vi "DRAFT3.vi"() -> ()   [LabVIEW 2021]
uses:
  <vilib>/Analysis/3filter.llb/Butterworth Filter (DBL).vi
  <vilib>/Analysis/NI_AALBase.lvlib
  <vilib>/ptbypt/NI_PtbyPt.lvlib
panel:
  out "Array Size":u32
  out "Elapsed time in ms":u32
  in  "stop":bool
  in  "error in (no error)":errorcluster
  out "error out":errorcluster
  in  "loop 1":i32
  out "Waveform Graph 6":dynamicdata(graph)
  out "Waveform Graph 5":dynamicdata(graph)
  out "Waveform Graph 4":dynamicdata(graph)
  out "Waveform Graph 3":dbl[](graph)
  out "Waveform Graph 2":dynamicdata(graph)
  in  "Boolean":bool
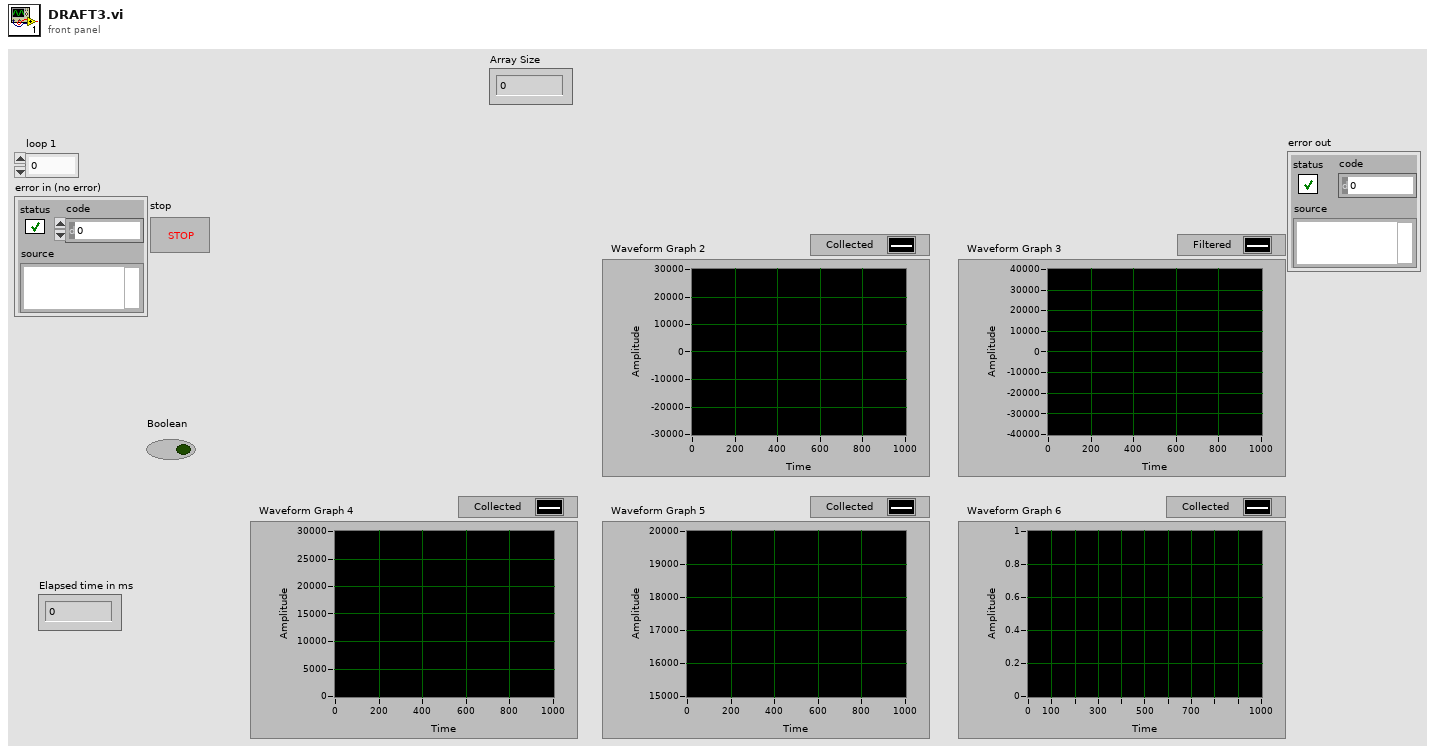
[diagram p1: front panel]
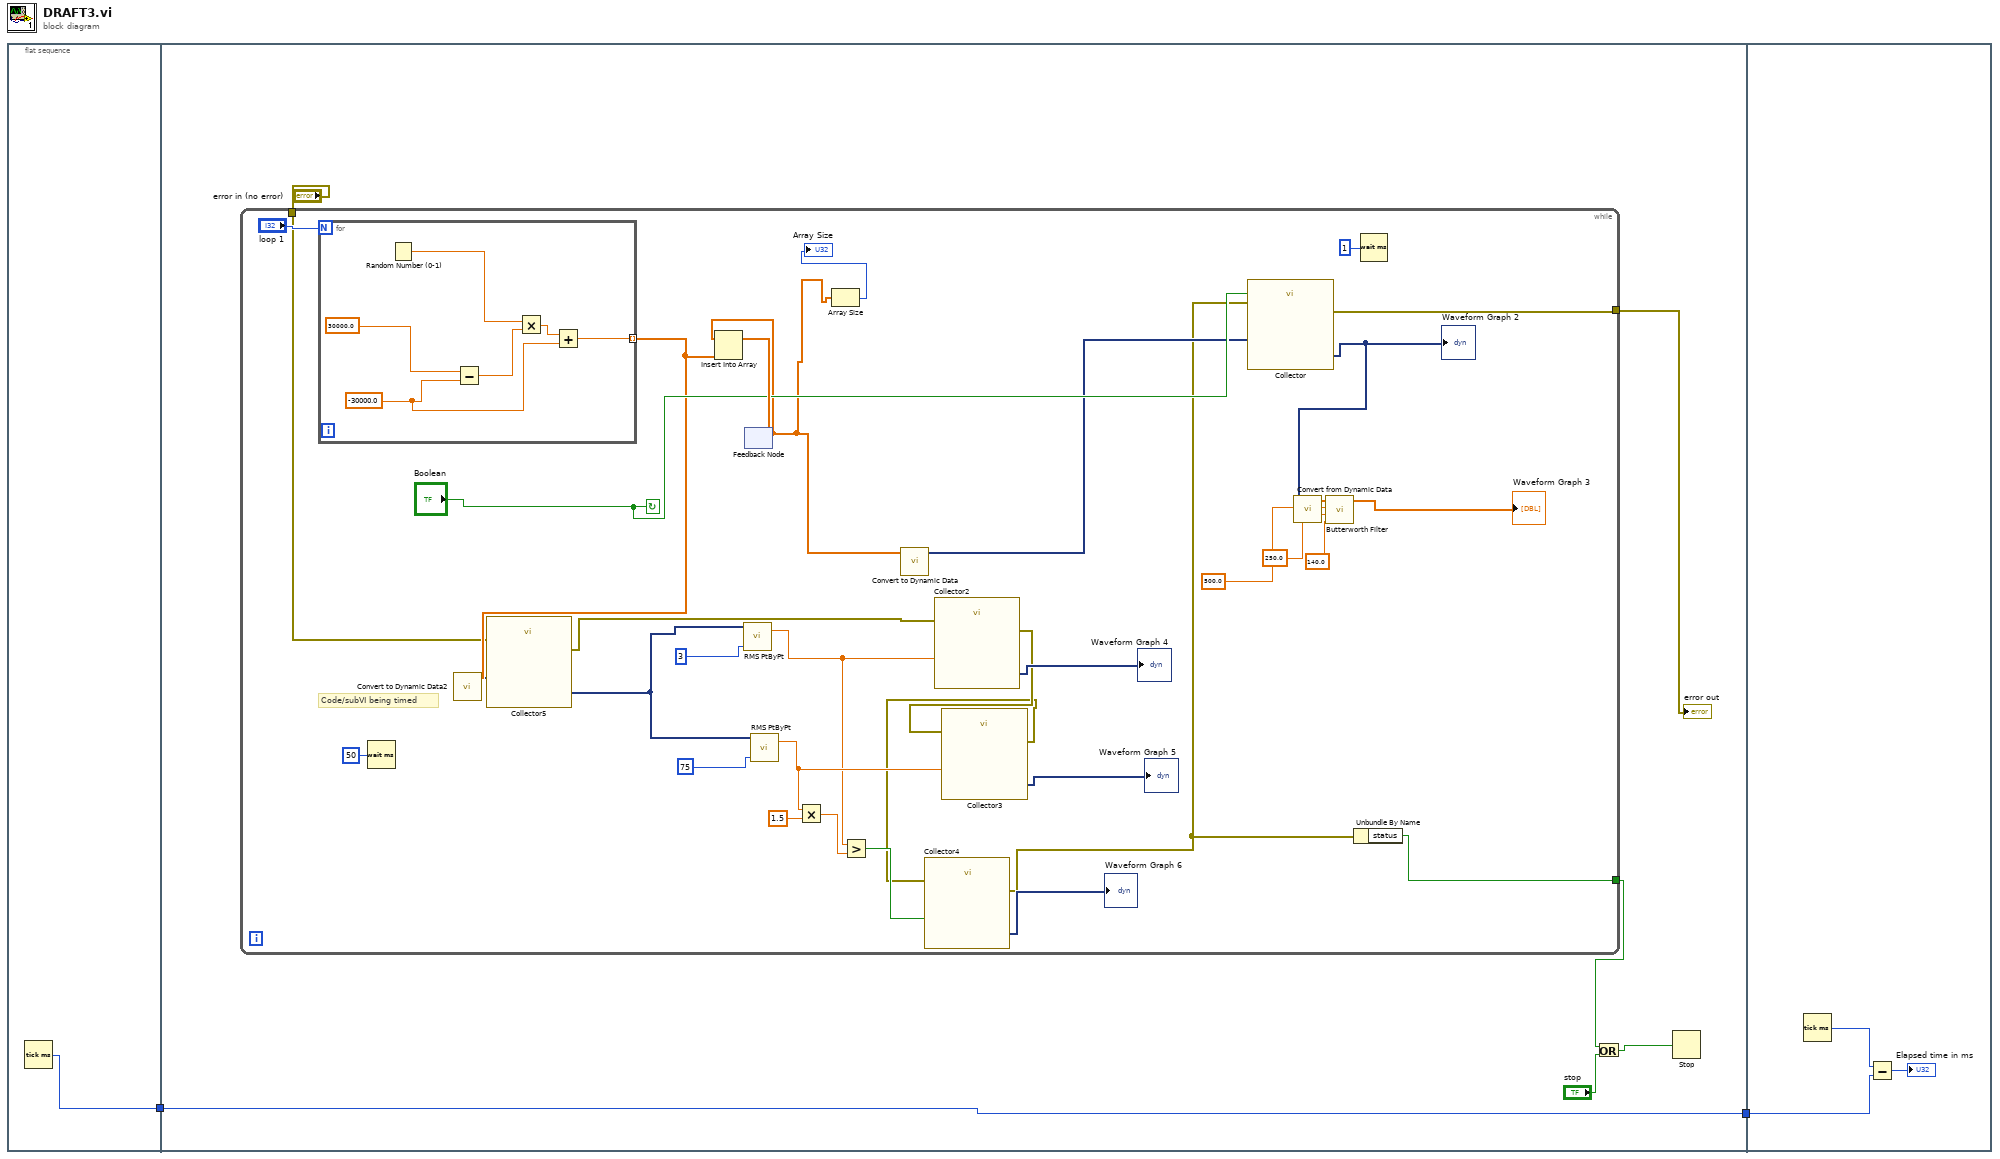
[diagram p0: block diagram]
diagram:
  n1 = flat-sequence {
    tunnel: [w3] -> w2
    tunnel: [w10] -> w1
    tunnel: w2 -> [w10]
    tunnel: w1 -> [w50]
    frame #0 {
      n2 = Tick Count (ms)() -> (millisecond timer value=w3:u32)
    }
    frame #1 {
      # "Code/subVI being timed"
      n3 = while {
        tunnel: "error in (no error)" -> [w19]
        tunnel: [w15] -> w7
        tunnel: [w13] -> w6
        stop <- "Boolean" continue-if-true
        n4 = for {
          N: "loop 1" -> [_]
          tunnel: [w44] -> w22 mode=indexing
          w46 = -30000.0 ("y")
          n5 = Random Number (0-1)() -> (number: 0 to 1=w45:dbl)
          n6 = Subtract(x=30000.0, y=w46) -> (x-y=w49:dbl)
          n7 = Multiply(x=w45, y=w49) -> (x*y=w48:dbl)
          n8 = Add(x=w48, y=w46) -> (x+y=w44:dbl)
        }
        n9 = call "Convert to Dynamic Data2"("Array"=w22) -> ("Dynamic Data Type"=w21:dynamicdata)  [unwired: 3 in]
        n10 = call "Collector5"("error in (no error)"=w19, "Signals"=w21) -> ("error out"=w18:errorcluster, "Collected Signals"=w20:dynamicdata)  [unwired: 8 in]
        n11 = call <vilib>:"RMS PtByPt.vi"("sample length"=3, "x"=w20) -> ("rms value"=w27:dbl)  [unwired: 2 in, 1 out]
        n12 = feedback #1() -> (w11:dbl[])  [unwired: 1 in]
        n13 = Insert Into Array(array=w11, new element=w22) -> (w43:dbl[])  [unwired: 1 in]
        n14 = feedback-in #1(w43) -> ()
        n15 = call <vilib>:"RMS PtByPt.vi"("sample length"=75, "x"=w20) -> ("rms value"=w30:dbl)  [unwired: 2 in, 1 out]
        n16 = Multiply(x=w30, y=1.5) -> (x*y=w28:dbl)
        n17 = Array Size(array=w11) -> (size(s)=→"Array Size":i32)
        n18 = Greater?(x=w27, y=w28) -> (0:w26:bool)
        n19 = call "Convert to Dynamic Data"("Array"=w11) -> ("Dynamic Data Type"=w33:dynamicdata)  [unwired: 3 in]
        n20 = call "Collector2"("error in (no error)"=w18, "Signals"=w27) -> ("error out"=w17:errorcluster, "Collected Signals"=→"Waveform Graph 4":dynamicdata)  [unwired: 8 in]
        n21 = call "Collector3"("error in (no error)"=w17, "Signals"=w30) -> ("error out"=w16:errorcluster, "Collected Signals"=→"Waveform Graph 5":dynamicdata)  [unwired: 8 in]
        n22 = call "Collector4"("error in (no error)"=w16, "Signals"=w26) -> ("error out"=w14:errorcluster, "Collected Signals"=→"Waveform Graph 6":dynamicdata)  [unwired: 8 in]
        n23 = call "Collector"("error in (no error)"=w14, "Enable"="Boolean", "Signals"=w33) -> ("error out"=w15:errorcluster, "Collected Signals"=w36:dynamicdata)  [unwired: 7 in]
        "Waveform Graph 2" <- w36
        n24 = call "Convert from Dynamic Data"("Dynamic Data Type"=w36) -> ("Array"=w38:dbl[])  [unwired: 3 in]
        n25 = call-poly <vilib>:"Butterworth Filter.vi"("low cutoff freq: fl"=140.0, "high cutoff freq: fh"=250.0, "sampling freq: fs"=500.0, "X"=w38) -> ("Filtered X"=→"Waveform Graph 3":dbl[])  [unwired: 4 in, 1 out]
        n26 = Unbundle By Name(w14) -> ("status"=w13:bool)
        n27 = Wait (ms)(milliseconds to wait=u32 1) -> ()  [unwired: 1 out]
      }
      "error out" <- w7
      n28 = Wait (ms)(milliseconds to wait=u32 50) -> ()  [unwired: 1 out]
      n29 = Or(x=w6, y="stop") -> (x .or. y?=w4:bool)
      n30 = Stop(stop? (T)=w4) -> ()
    }
    frame #2 {
      n31 = Tick Count (ms)() -> (millisecond timer value=w52:u32)
      n32 = Subtract(x=w52, y=w50) -> (x-y=→"Elapsed time in ms":u32)
    }
  }
